vi "Main.vi"() -> ()   [LabVIEW 2014]
doc: "This template is for the Queued Message Handler design pattern.\n\nThe Event Handling Loop generates messages based on user interface actions.\n\nThe Message Handling Loop processes messages generated by the Event Handling Loop, or by other messages. The messages are string values, so new messages can be added easily to the Message Cases case structure in the Message Handling Loop. Each message cluster can also provide an optional value for Message Data, which is a variant that can be converted to whatever message-specific data is required."
uses:
  Controls/UI Data.ctl
  QMH/Message Queue/Message Queue.lvlib
  <vilib>/Utility/error.llb/Error Cluster From Error Code.vi
  QMH/User Event - Stop/User Event - Stop.lvlib
  QMH/Message Queue/Enqueue Message (Single).vi
  <vilib>/ErrorRing/Error Ring.xnode
  Controls/Control 2.ctl
panel:
  in  "Template Action 3":bool
  in  "Array - String":string[](array[string])=["Template #1", "Template #2", "Filter Wheel", "Live"]
  in  "Template Action 1":dbl
  in  "Template Action 2":bool
  out "Status array":T1
  out "Current task":string="\"Exit\" button pressed"
  in  "Exit":bool=TRUE
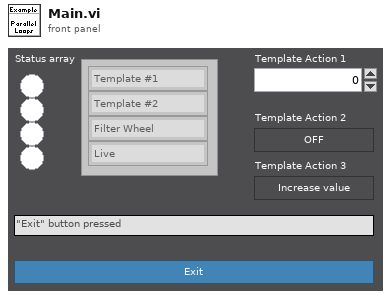
[diagram p1: front panel]
types:
  T1 = typedef "Control 2.ctl" = bool[]
  T2 = typedef "UI Data.ctl" = cluster{"Boolean <Replace Me>":bool, "String <Replace Me>":string, "Numeric <Replace Me>":dbl, "Data Display Ref":refnum<vi>, "Exit Button Ref":refnum<vi>}
  T3 = typedef "Message Queue.lvlib/All Message Queues.ctl" = cluster{"UI":refnum<queue>, "Template loop":refnum<queue>, "Template loop 2":refnum<queue>}
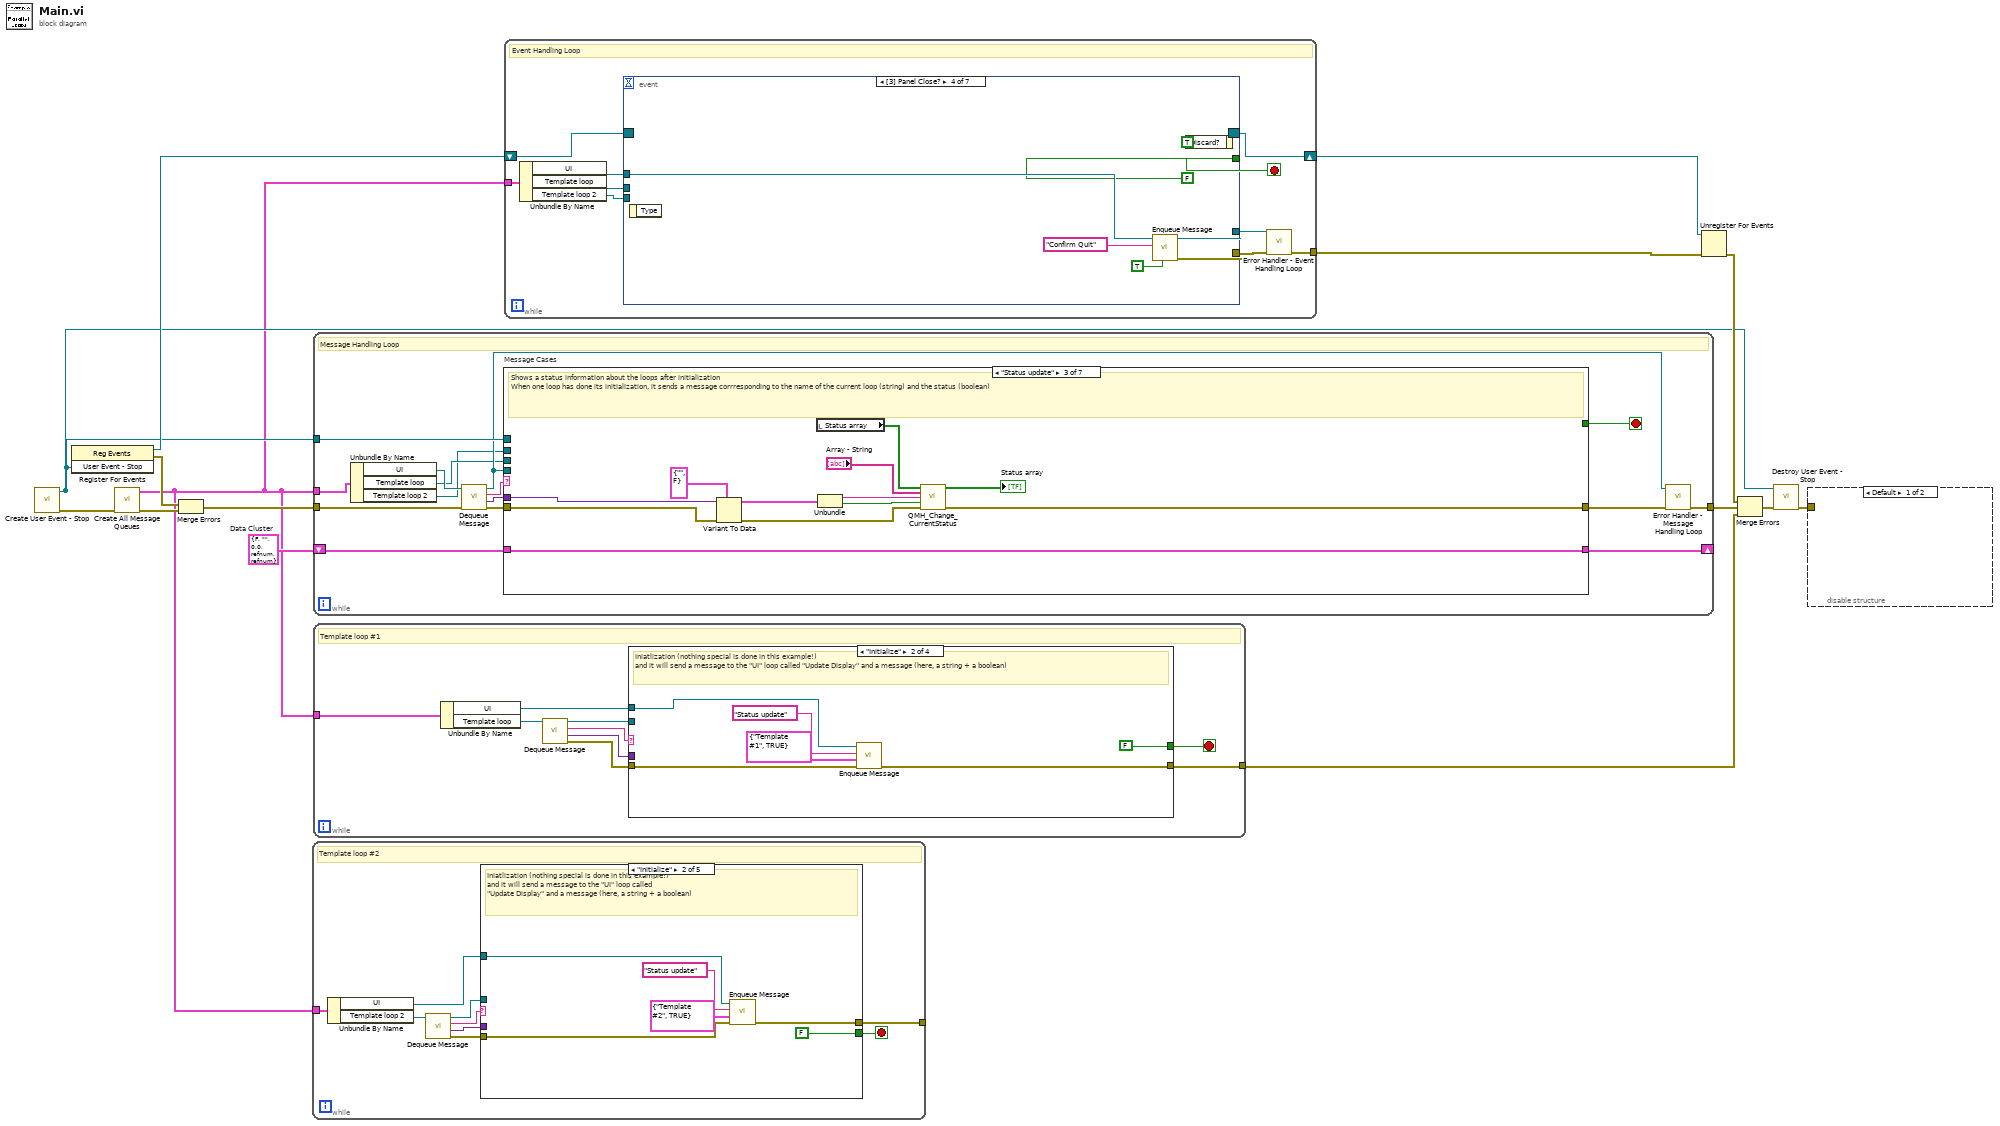
[diagram p0: block diagram]
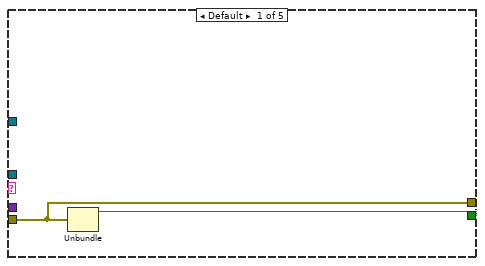
[diagram p2: hidden frame]
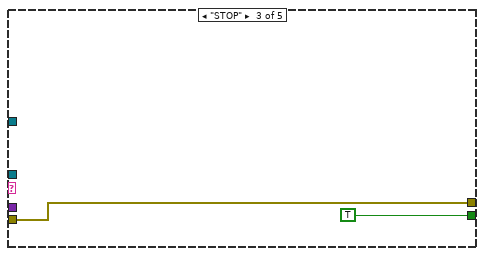
[diagram p3: hidden frame]
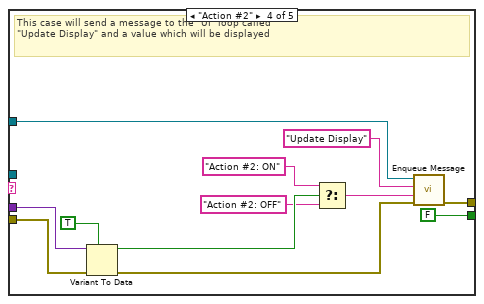
[diagram p4: hidden frame]
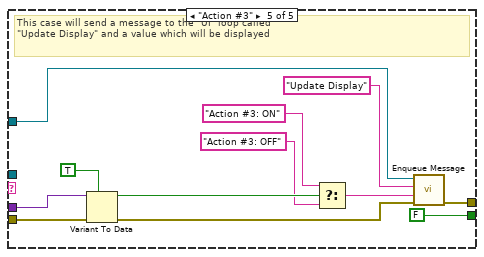
[diagram p5: hidden frame]
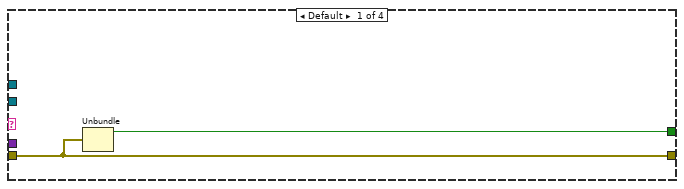
[diagram p6: hidden frame]
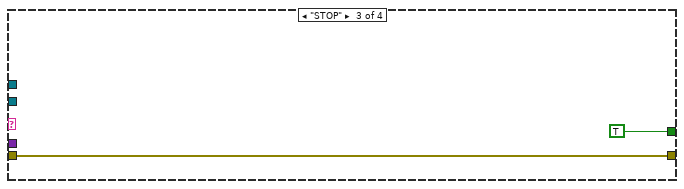
[diagram p7: hidden frame]
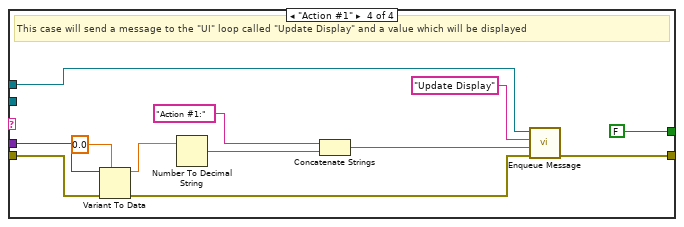
[diagram p8: hidden frame]
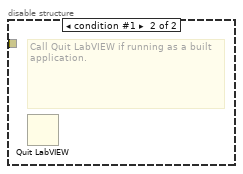
[diagram p9: hidden frame]
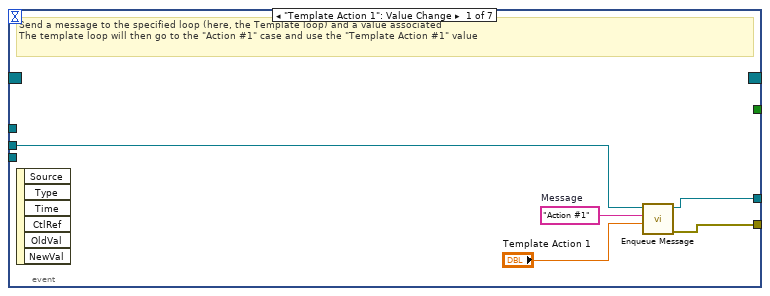
[diagram p10: hidden frame]
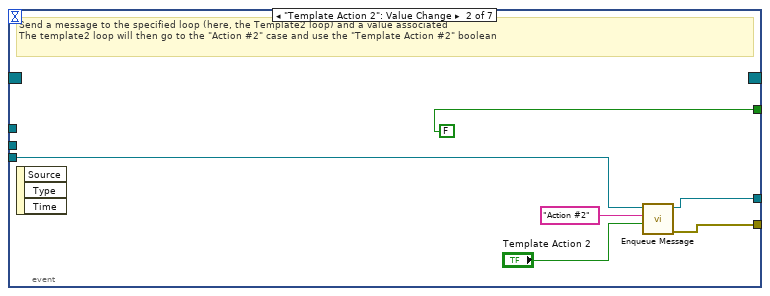
[diagram p11: hidden frame]
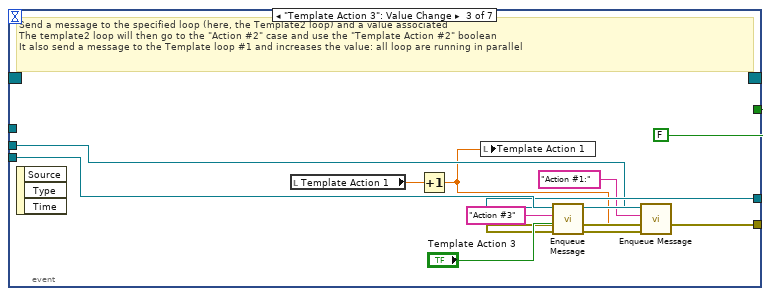
[diagram p12: hidden frame]
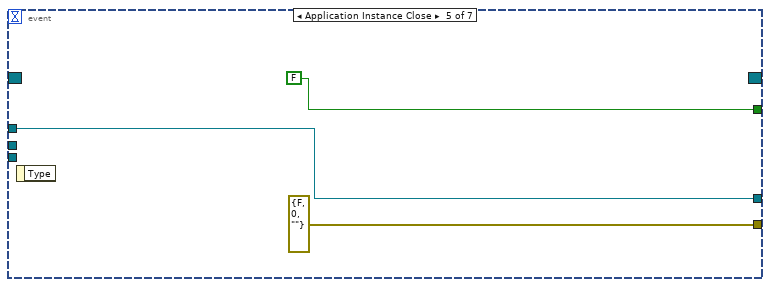
[diagram p13: hidden frame]
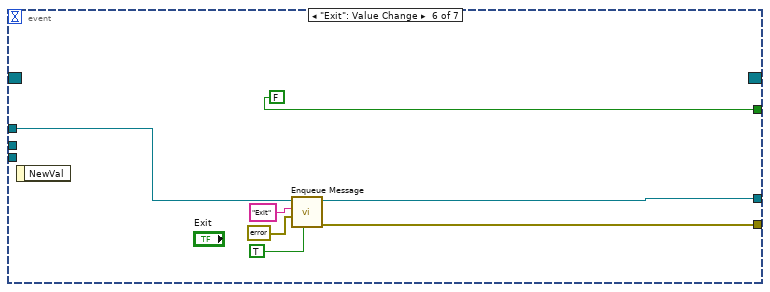
[diagram p14: hidden frame]
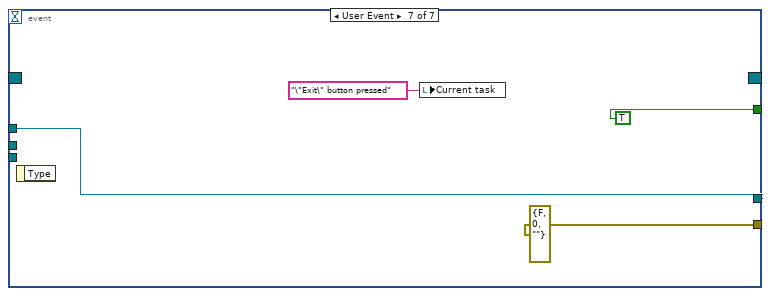
[diagram p15: hidden frame]
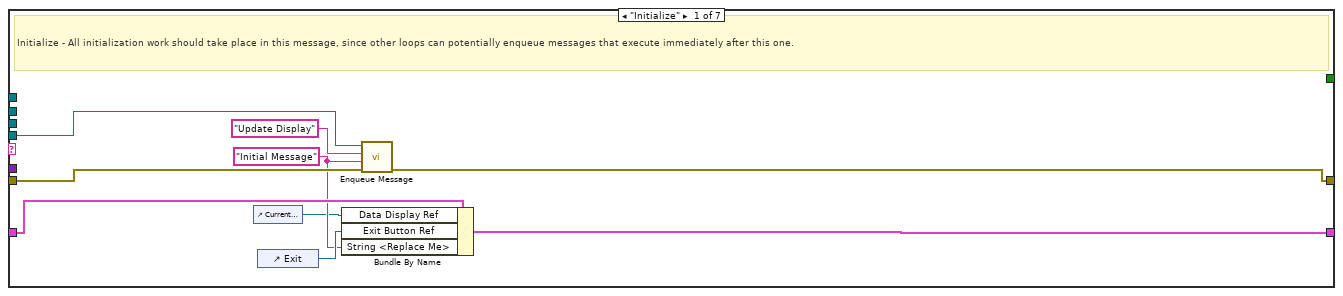
[diagram p16: hidden frame]
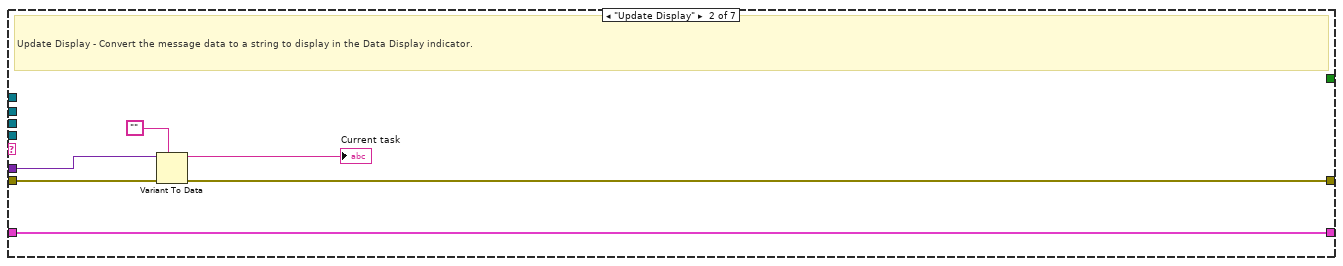
[diagram p17: hidden frame]
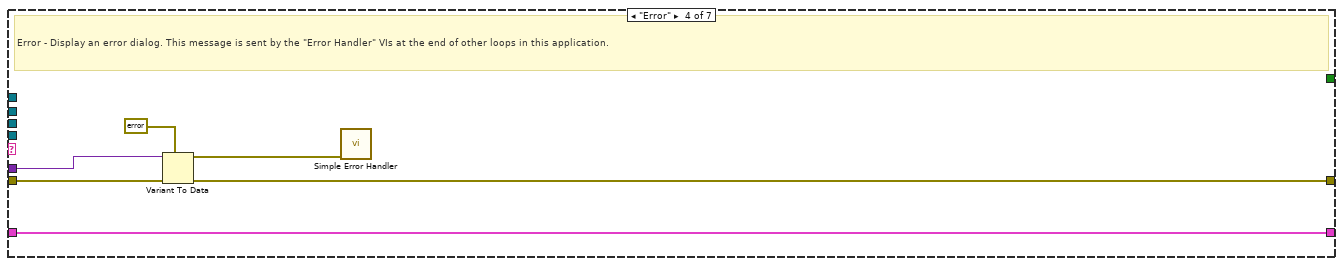
[diagram p18: hidden frame]
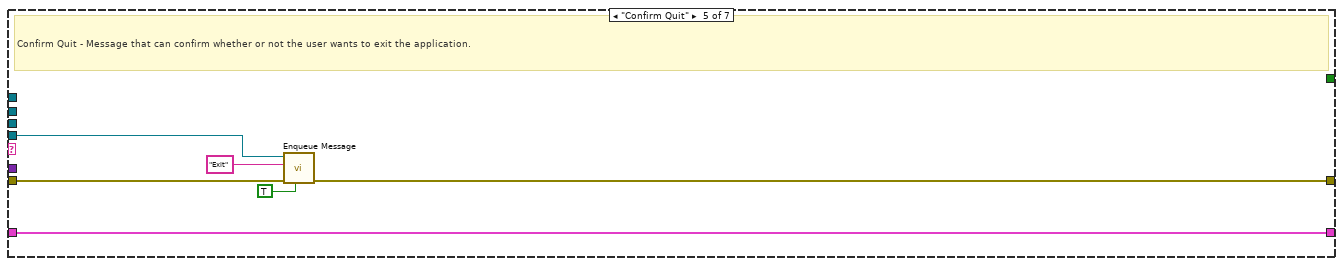
[diagram p19: hidden frame]
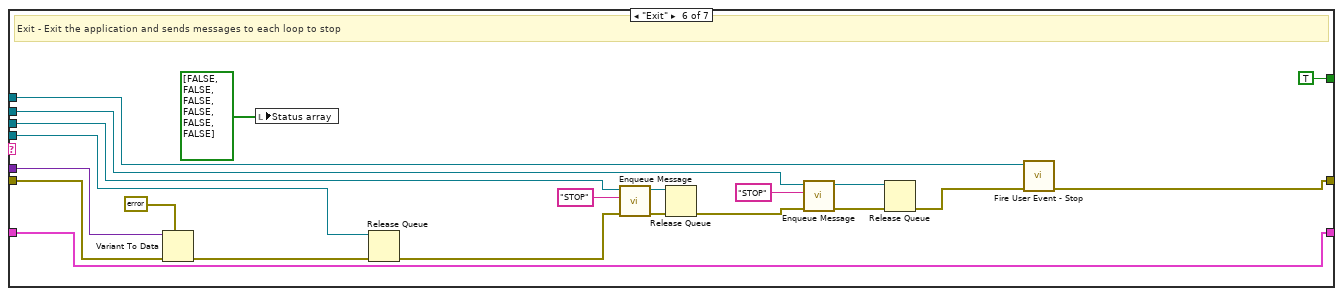
[diagram p20: hidden frame]
diagram:
  w3 = T2 {"Boolean <Replace Me>"=FALSE, "String <Replace Me>"="", "Numeric <Replace Me>"=0.0, "Data Display Ref"=refnum, "Exit Button Ref"=refnum}  # Data Cluster
  n1 = call "Create User Event - Stop.vi"() -> ("error out"=w13:errorcluster, "User Event - Stop"=w6:refnum<user-event>)  [unwired: 10 in]
  n2 = register-events(w6) -> (reference out=w7:refnum<event-registration>, error out=w4:errorcluster)  [unwired: 2 in]
  n3 = call "Create All Message Queues.vi"("error in (no error)"=w13) -> ("error out"=w15:errorcluster, "Message Queues out"=w1:T3)  [unwired: 9 in]
  n4 = Merge Errors(w4, w15) -> (w5:errorcluster)
  n5 = while {
    tunnel: [w20] -> _
    tunnel: w1 -> [w18]
    stop <- w21 stop-if-true
    # "Template loop #2"
    n6 = Unbundle By Name(w18) -> ("UI"=w17:refnum<queue>, "Template loop 2"=w16:refnum<queue>)
    n7 = call "Dequeue Message.vi"("Message Queue"=w16) -> ("error out"=w24:errorcluster, "Message Data"=w22:variant, "Message"=w23:string, "dup Message Queue"=w19:refnum<queue>)  [unwired: 7 in]
    n8 = case shown="\"Initialize\"" w23 {
      tunnel: w24 -> [w26 w32 w33 w42 w54]
      tunnel: w22 -> [_ _ _ w40 w52]
      tunnel: w17 -> [_ w31 _ w44 w56]
      tunnel: [w25 FALSE ("status") TRUE FALSE ("status") FALSE ("status")] -> w21
      tunnel: [w26 w28 w33 w43 w55] -> w20
      tunnel: w19 -> [_ _ _ _ _]
      frame Default {
        n9 = Unbundle(w26) -> ("status"=w25:bool)  [unwired: 2 out]
      }
      frame "Initialize" {
        # "Iniatlization (nothing special is done in this example!)\nand it will send a message to the \"UI\" loop called\n\"Update Display\" and a message (here, a string + a boolean)"
        n10 = call-poly "Enqueue Message.vi"("error in (no error)"=w32, "Message Data"=cluster{string, bool} {"Template #2", TRUE}, "Message"="Status update", "Message Queue"=w31) -> ("error out"=w28:errorcluster)  [unwired: 6 in, 1 out]
      }
      frame "STOP" {
      }
      frame "Action #2" {
        # "This case will send a message to the \"UI\" loop called\n\"Update Display\" and a value which will be displayed"
        n11 = Variant To Data(error in=w42, type=TRUE, Variant=w40) -> (data=w38:bool, error out=w41:errorcluster)
        n12 = Select(t="Action #2: ON" ("Message"), s=w38, f="Action #2: OFF" ("Message")) -> (s? t:f=w35:string)
        n13 = call-poly "Enqueue Message.vi"("error in (no error)"=w41, "Message Data"=w35, "Message"="Update Display", "Message Queue"=w44) -> ("error out"=w43:errorcluster)  [unwired: 6 in, 1 out]
      }
      frame "Action #3" {
        # "This case will send a message to the \"UI\" loop called\n\"Update Display\" and a value which will be displayed"
        n14 = Variant To Data(error in=w54, type=TRUE, Variant=w52) -> (data=w50:bool, error out=w53:errorcluster)
        n15 = Select(t="Action #3: ON" ("Message"), s=w50, f="Action #3: OFF" ("Message")) -> (s? t:f=w47:string)
        n16 = call-poly "Enqueue Message.vi"("error in (no error)"=w53, "Message Data"=w47, "Message"="Update Display", "Message Queue"=w56) -> ("error out"=w55:errorcluster)  [unwired: 6 in, 1 out]
      }
    }
  }
  n17 = while {
    shift-right: [w72] -> _
    shift-left: w3 -> [w73]
    tunnel: w6 -> [w70]
    tunnel: w5 -> [w69]
    tunnel: [w64] -> w14
    tunnel: w1 -> [w62]
    stop <- w71 stop-if-true
    # "Message Handling Loop"
    n18 = Unbundle By Name(w62) -> ("UI"=w61:refnum<queue>, "Template loop"=w60:refnum<queue>, "Template loop 2"=w59:refnum<queue>)
    n19 = call "Dequeue Message.vi"("error in (no error)"=w69, "Message Queue"=w61) -> ("error out"=w68:errorcluster, "Message Data"=w66:variant, "Message"=w67:string, "dup Message Queue"=w65:refnum<queue>)  [unwired: 6 in]
    n20 = case "Message Cases" shown="\"Status update\"" w67 {
      selector: w67 -> [_ _ _ _ _ _ w134]
      tunnel: w65 -> [w76 _ _ _ w110 w125 _]
      tunnel: w68 -> [w81 w87 w97 w106 w112 w126 _]
      tunnel: [w82 w84 w96 w101 w107 w121 w135] -> w63
      tunnel: w73 -> [w80 w88 w100 w105 w111 w133 w136]
      tunnel: [w79 w88 w100 w105 w111 w133 w136] -> w72
      tunnel: [_ _ _ _ _ TRUE _] -> w71
      tunnel: w66 -> [_ w86 w95 w104 _ w129 _]
      tunnel: w70 -> [_ _ _ _ _ w131 _]
      tunnel: w60 -> [_ _ _ _ _ w124 _]
      tunnel: w59 -> [_ _ _ _ _ w113 _]
      frame "Initialize" {
        w75 = "Initial Message" ("Initial Message")
        # "Initialize - All initialization work should take place in this message, since other loops can potentially enqueue messages that execute immediately after this one."
        n21 = control-ref of="Current task"() -> (w74:refnum<vi>)
        n22 = control-ref of="Exit"() -> (w78:refnum<vi>)
        n23 = Bundle By Name(cluster=w80, "Data Display Ref"=w74, "Exit Button Ref"=w78, "String <Replace Me>"=w75) -> (w79:T2)
        n24 = call-poly "Enqueue Message.vi"("error in (no error)"=w81, "Message Data"=w75, "Message"="Update Display", "Message Queue"=w76) -> ("error out"=w82:errorcluster)  [unwired: 6 in, 1 out]
      }
      frame "Update Display" {
        # "Update Display - Convert the message data to a string to display in the Data Display indicator."
        n25 = Variant To Data(error in=w87, type="", Variant=w86) -> (data=→"Current task":string, error out=w84:errorcluster)
      }
      frame "Status update" {
        # "Shows a status information about the loops after initialization\nWhen one loop has done its initialization, it sends a message corrresponding to the name of the current loop (string) and the status (boolean)"
        n26 = Variant To Data(error in=w97, type=cluster{string, bool} {"", FALSE}, Variant=w95) -> (data=w92:cluster{string, bool}, error out=w94:errorcluster)
        n27 = local read "Status array"() -> (w98:T1)
        n28 = Unbundle(w92) -> (w91:string, w90:bool)
        n29 = call "QMH_Change_CurrentStatus.vi"("Status array in"=w98, "Array - String"="Array - String", "String to find"=w91, "New status"=w90, "error in (no error)"=w94) -> ("Status array out"=→"Status array":T1, "error out"=w96:errorcluster)  [unwired: 9 in]
      }
      frame "Error" {
        # "Error - Display an error dialog. This message is sent by the \"Error Handler\" VIs at the end of other loops in this application."
        n30 = Variant To Data(error in=w106, type=errorcluster {"status"=FALSE, "code"=0, "source"=""} ("error constant"), Variant=w104) -> (data=w102:errorcluster, error out=w101:errorcluster)
        n31 = call <vilib>:"Simple Error Handler.vi"("error in (no error)"=w102) -> ()  [unwired: 4 in, 5 out]
      }
      frame "Confirm Quit" {
        # "Confirm Quit - Message that can confirm whether or not the user wants to exit the application."
        n32 = call-poly "Enqueue Message.vi"("Priority Message? (F)"=TRUE, "error in (no error)"=w112, "Message"="Exit", "Message Queue"=w110) -> ("error out"=w107:errorcluster)  [unwired: 6 in, 1 out]
      }
      frame "Exit" {
        # "Exit - Exit the application and sends messages to each loop to stop"
        n33 = Variant To Data(error in=w126, type=errorcluster {"status"=FALSE, "code"=0, "source"=""} ("error constant"), Variant=w129) -> (error out=w122:errorcluster)  [unwired: 1 out]
        n34 = local write "Status array"(T1 [FALSE, FALSE, FALSE, FALSE, FALSE, FALSE] ("Status array")) -> ()
        n35 = Release Queue(queue=w125, error in (no error)=w122) -> (error out=w119:errorcluster)  [unwired: 1 in, 2 out]
        n36 = call-poly "Enqueue Message.vi"("error in (no error)"=w119, "Message"="STOP", "Message Queue"=w124) -> ("error out"=w128:errorcluster, "dup Message Queue"=w127:refnum<queue>)  [unwired: 7 in]
        n37 = Release Queue(queue=w127, error in (no error)=w128) -> (error out=w115:errorcluster)  [unwired: 1 in, 2 out]
        n38 = call-poly "Enqueue Message.vi"("error in (no error)"=w115, "Message"="STOP", "Message Queue"=w113) -> ("error out"=w116:errorcluster, "dup Message Queue"=w117:refnum<queue>)  [unwired: 7 in]
        n39 = Release Queue(queue=w117, error in (no error)=w116) -> (error out=w114:errorcluster)  [unwired: 1 in, 2 out]
        n40 = call "Fire User Event - Stop.vi"("error in (no error)"=w114, "User Event - Stop"=w131) -> ("error out"=w121:errorcluster)  [unwired: 9 in]
      }
      frame Default {
        # "'Default' case only runs if there is a message that isn't defined in any of the other cases.  Output a programming error."
        n41 = xnode "Error Ring"("parameter 0"=w134) -> ("error out"=w135:errorcluster)
      }
    }
    n42 = call "Error Handler - Message Handling Loop.vi"("error in (no error)"=w63, "Message Queue"=w65) -> ("dup error in"=w64:errorcluster)  [unwired: 8 in, 1 out]
  }
  n43 = while {
    tunnel: [w148] -> w2
    tunnel: w1 -> [w146]
    stop <- w149 stop-if-true
    # "Template loop #1"
    n44 = Unbundle By Name(w146) -> ("UI"=w145:refnum<queue>, "Template loop"=w144:refnum<queue>)
    n45 = call "Dequeue Message.vi"("Message Queue"=w144) -> ("error out"=w152:errorcluster, "Message Data"=w150:variant, "Message"=w151:string, "dup Message Queue"=w147:refnum<queue>)  [unwired: 7 in]
    n46 = case shown="\"Initialize\"" w151 {
      tunnel: w152 -> [w154 w160 w161 w170]
      tunnel: w150 -> [_ _ _ w168]
      tunnel: w145 -> [_ w159 _ w172]
      tunnel: [w153 FALSE ("status") TRUE FALSE ("status")] -> w149
      tunnel: [w154 w156 w161 w171] -> w148
      tunnel: w147 -> [_ _ _ _]
      frame Default {
        n47 = Unbundle(w154) -> ("status"=w153:bool)  [unwired: 2 out]
      }
      frame "Initialize" {
        # "Iniatlization (nothing special is done in this example!)\nand it will send a message to the \"UI\" loop called \"Update Display\" and a message (here, a string + a boolean)"
        n48 = call-poly "Enqueue Message.vi"("error in (no error)"=w160, "Message Data"=cluster{string, bool} {"Template #1", TRUE}, "Message"="Status update", "Message Queue"=w159) -> ("error out"=w156:errorcluster)  [unwired: 6 in, 1 out]
      }
      frame "STOP" {
      }
      frame "Action #1" {
        # "This case will send a message to the \"UI\" loop called \"Update Display\" and a value which will be displayed"
        n49 = Variant To Data(error in=w170, type=0.0, Variant=w168) -> (data=w165:dbl, error out=w169:errorcluster)
        n50 = Number To Decimal String(number=w165) -> (decimal integer string=w164:string)  [unwired: 1 in]
        n51 = Concatenate Strings("Action #1:" ("Message"), w164) -> (w163:string)
        n52 = call-poly "Enqueue Message.vi"("error in (no error)"=w169, "Message Data"=w163, "Message"="Update Display", "Message Queue"=w172) -> ("error out"=w171:errorcluster)  [unwired: 6 in, 1 out]
      }
    }
  }
  n53 = while {
    shift-right: [w183] -> w10
    shift-left: w7 -> [w184]
    tunnel: [w179] -> w8
    tunnel: w1 -> [w176]
    stop <- w181 stop-if-true
    # "Event Handling Loop"
    n54 = Unbundle By Name(w176) -> ("UI"=w178:refnum<queue>, "Template loop"=w177:refnum<queue>, "Template loop 2"=w175:refnum<queue>)
    n55 = event shown="[3] Panel Close?" {
      selector: w184 -> [_ _ _ _ _ _ _]
      dyn-events: [_ _ _ _ _ _ _] -> w183
      timeout: _ -> [_ _ _ _ _ _ _]
      tunnel: [_ FALSE ("Discard?") FALSE ("Discard?") FALSE ("Discard?") FALSE ("Discard?") FALSE ("Discard?") TRUE ("Discard?")] -> w181
      tunnel: w178 -> [_ _ _ w212 w216 w223 w227]
      tunnel: [w188 w194 w201 w211 errorcluster {"status"=FALSE, "code"=0, "source"=""} ("error out") w217 errorcluster {"status"=FALSE, "code"=0, "source"=""} ("error out")] -> w182
      tunnel: [w187 w195 w200 w210 w216 w222 w227] -> w180
      tunnel: w177 -> [w185 _ w199 _ _ _ _]
      tunnel: w175 -> [_ w190 w203 _ _ _ _]
      event "Template Action 1": Value Change {
        w189 = "Action #1"  # Message
        # "Send a message to the specified loop (here, the Template loop) and a value associated\nThe template loop will then go to the \"Action #1\" case and use the \"Template Action #1\" value"
        n56 = event-data() -> ()  [unwired: 1 in, 6 out]
        n57 = call-poly "Enqueue Message.vi"("Message Data"="Template Action 1", "Message"=w189, "Message Queue"=w185) -> ("error out"=w188:errorcluster, "dup Message Queue"=w187:refnum<queue>)  [unwired: 7 in]
      }
      event "Template Action 2": Value Change {
        # "Send a message to the specified loop (here, the Template2 loop) and a value associated\nThe template2 loop will then go to the \"Action #2\" case and use the \"Template Action #2\" boolean"
        n58 = event-data() -> ()  [unwired: 1 in, 3 out]
        n59 = call-poly "Enqueue Message.vi"("Message Data"="Template Action 2", "Message"="Action #2", "Message Queue"=w190) -> ("error out"=w194:errorcluster, "dup Message Queue"=w195:refnum<queue>)  [unwired: 7 in]
      }
      event "Template Action 3": Value Change {
        # "Send a message to the specified loop (here, the Template2 loop) and a value associated\nThe template2 loop will then go to the \"Action #2\" case and use the \"Template Action #2\" boolean\nIt also send a message to the Template loop #1 and increases the value: all loop are running in parallel"
        n60 = event-data() -> ()  [unwired: 1 in, 3 out]
        n61 = local read "Template Action 1"() -> (w197:dbl)
        n62 = Increment(x=w197) -> (x+1=w196:dbl)
        n63 = local write "Template Action 1"(w196) -> ()
        n64 = call-poly "Enqueue Message.vi"("Message Data"="Template Action 3", "Message"="Action #3", "Message Queue"=w203) -> ("error out"=w202:errorcluster)  [unwired: 7 in, 1 out]
        n65 = call-poly "Enqueue Message.vi"("error in (no error)"=w202, "Message Data"=w196, "Message"="Action #1:", "Message Queue"=w199) -> ("error out"=w201:errorcluster, "dup Message Queue"=w200:refnum<queue>)  [unwired: 6 in]
      }
      event Panel Close? {
        n66 = event-data() -> ()  [unwired: 1 in, 1 out]
        n67 = call-poly "Enqueue Message.vi"("Priority Message? (F)"=TRUE, "Message"="Confirm Quit", "Message Queue"=w212) -> ("error out"=w211:errorcluster, "dup Message Queue"=w210:refnum<queue>)  [unwired: 7 in]
        n68 = event-data("Discard?"=TRUE) -> ()  [unwired: 1 in, 1 out]
      }
      event Application Instance Close {
        n69 = event-data() -> ()  [unwired: 1 in, 1 out]
      }
      event "Exit": Value Change {
        n70 = event-data() -> ()  [unwired: 1 in, 1 out]
        n71 = call-poly "Enqueue Message.vi"("Priority Message? (F)"=TRUE, "Message Data"=errorcluster {"status"=FALSE, "code"=0, "source"=""} ("error constant"), "Message"="Exit", "Message Queue"=w223) -> ("error out"=w217:errorcluster, "dup Message Queue"=w222:refnum<queue>)  [unwired: 6 in]
      }
      event User Event {
        n72 = event-data() -> ()  [unwired: 1 in, 1 out]
        n73 = local write "Current task"("\"Exit\" button pressed" ("VI Stopped")) -> ()
      }
    }
    n74 = call "Error Handler - Event Handling Loop.vi"("error in (no error)"=w182, "Message Queue"=w180) -> ("dup error in"=w179:errorcluster)  [unwired: 8 in, 1 out]
  }
  n75 = Unregister For Events(event registration refnum=w10, error in=w8) -> (error out=w11:errorcluster)
  n76 = Merge Errors(w11, w14, w2) -> (w12:errorcluster)
  n77 = call "Destroy User Event - Stop.vi"("error in (no error)"=w12, "User Event - Stop"=w6) -> ("error out"=w9:errorcluster)  [unwired: 9 in]
  n78 = disable-structure shown="Default" {
    disable-tunnel: w9 -> [_ _]
    frame condition #0 (active) {
    }
    frame condition #1 {
      # "Call Quit LabVIEW if running as a built application."
      n79 = Quit LabVIEW() -> ()  [unwired: 1 in]
    }
  }
